vi "SCAN IM Stage Engine.vi"(0 "Notifier Name":string, 11 "COM Port":string[](array[string])) -> ()   [LabVIEW 2020]
uses:
  Stages Controls/Stage XY Control.ctl
  Stages Controls/Stage Status.ctl
  Stages Controls/Stage Notifier Element.ctl
  Stages Controls/Stage Actions.ctl
  <userlib>/Tango_DLL/Tango_DLL.lvlib
panel:
  out "Status":T1
  in  "Quit":bool
  in  "XY Control":T2
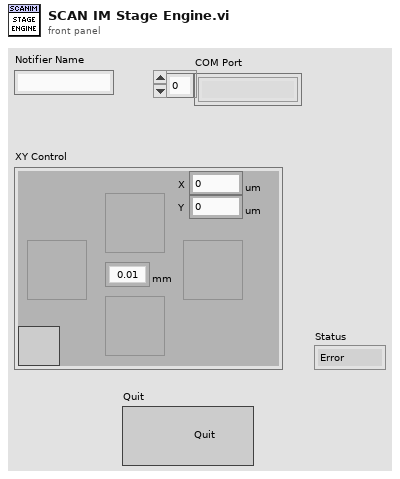
[diagram p1: front panel]
types:
  T1 = typedef "Stage Status.ctl" = enum16{"Error", "Abort", "Busy", "On Target"}
  T2 = typedef "Stage XY Control.ctl" = cluster{"Left":bool, "Right":bool, "Up":bool, "Down":bool, "Home":bool, "StageStep":enum16{"0.01", "0.02", "0.05", "0.1", "0.5", "1", "2", "5", "10", "20", "50", "100", "500", "1000", "2000", "5000"}, "Y":dbl, "X":dbl}
  T3 = typedef "Stage Notifier Element.ctl" = cluster{"Action":T4, "Axis":bool[], "Setpoint":dbl[], "Velocity":dbl, "Cmd Recvd?":bool, "Position":dbl[], "Status":T1, "Misc":variant}
  T4 = typedef "Stage Actions.ctl" = enum16{"Get Position", "MVR", "MOVE", "HALT", "ONTARGET", "ERROR", "REFERENCE", "INIT", "VELOCITY", "STATUS", "EXIT", "HOME", "ZEROPOS", "NANOPOS", "ANALOG", "QUIT"}
  T5 = cluster{"Left":bool, "Right":bool, "Up":bool, "Down":bool, "Home":bool, "StageStep":bool, "Y":bool, "X":bool}
  T6 = enum16{"0.01", "0.02", "0.05", "0.1", "0.5", "1", "2", "5", "10", "20", "50", "100", "500", "1000", "2000", "5000"}
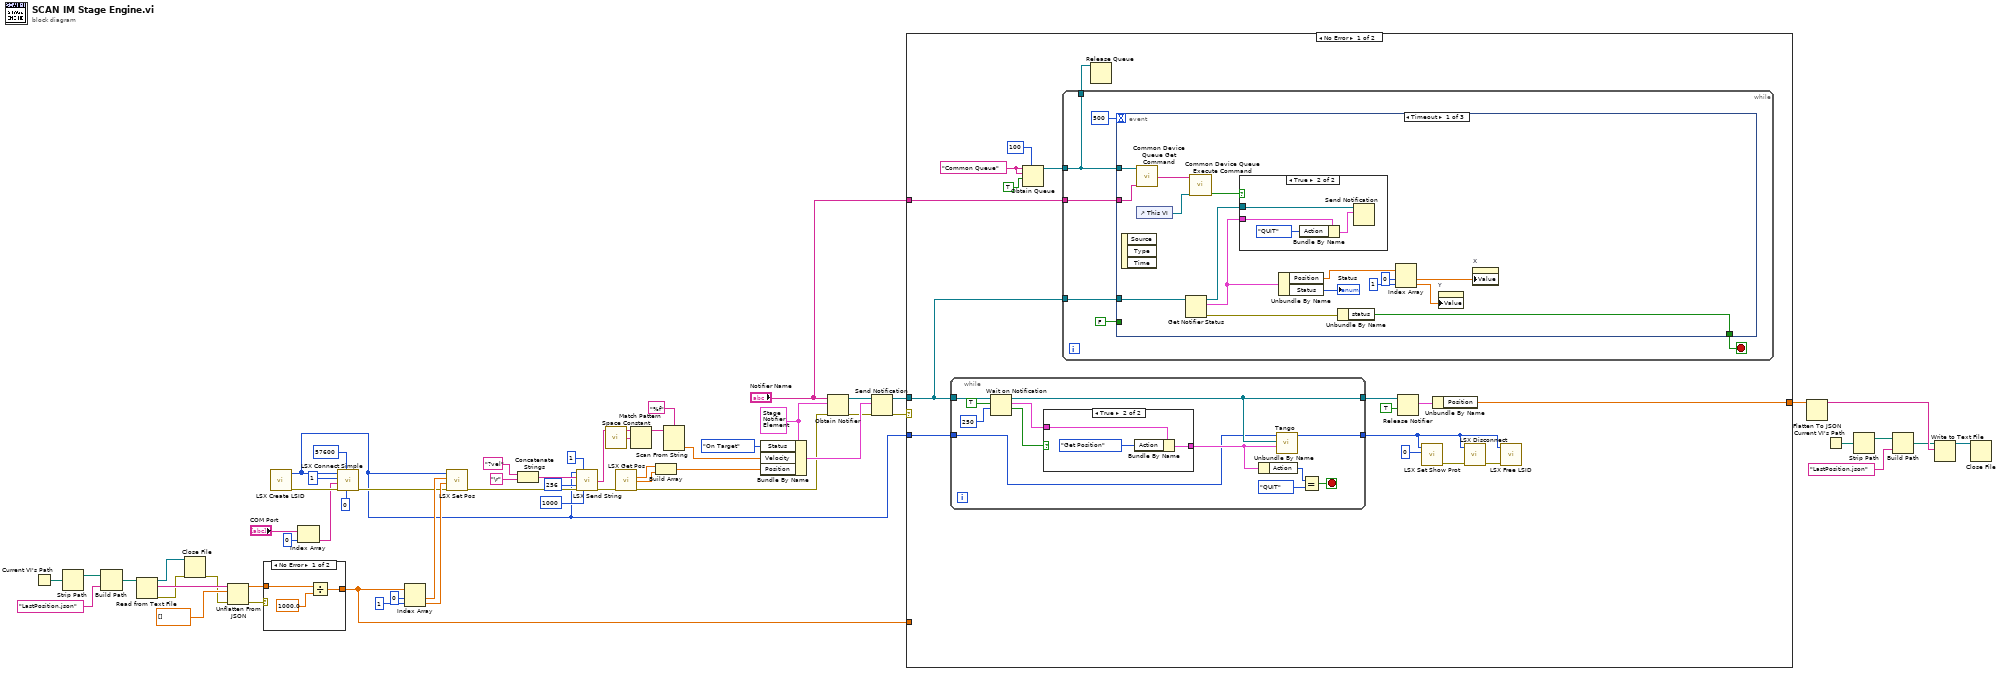
[diagram p0: block diagram]
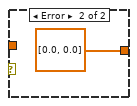
[diagram p2: hidden frame]
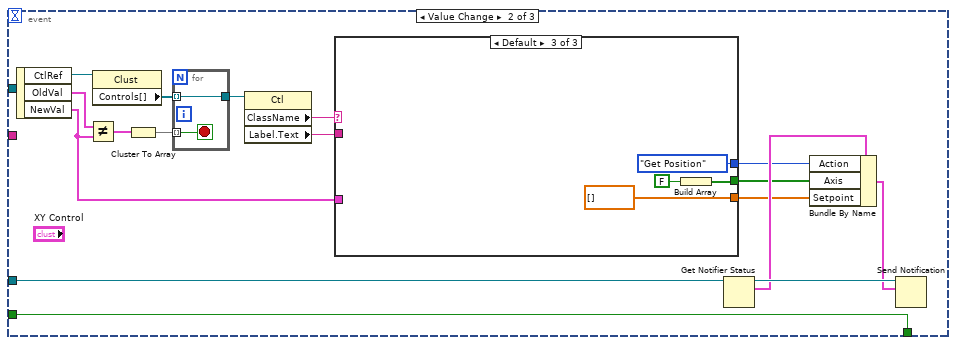
[diagram p5: hidden frame]
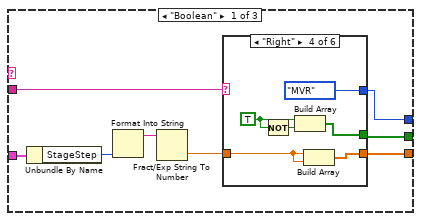
[diagram p6: hidden frame]
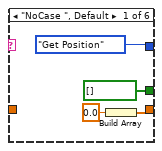
[diagram p7: hidden frame]
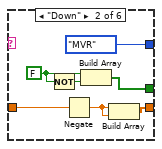
[diagram p8: hidden frame]
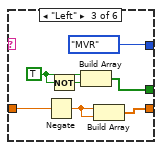
[diagram p9: hidden frame]
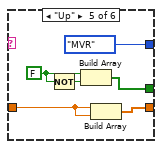
[diagram p10: hidden frame]
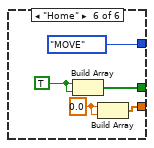
[diagram p11: hidden frame]
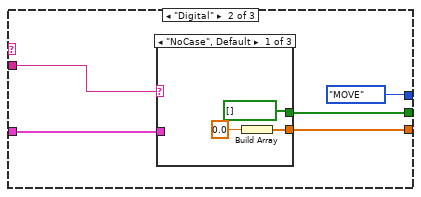
[diagram p12: hidden frame]
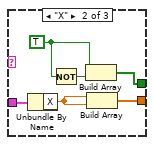
[diagram p13: hidden frame]
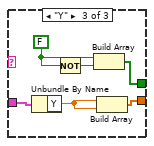
[diagram p14: hidden frame]
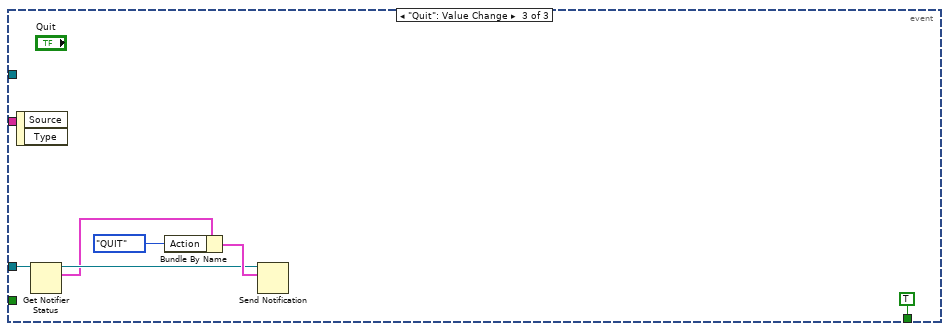
[diagram p15: hidden frame]
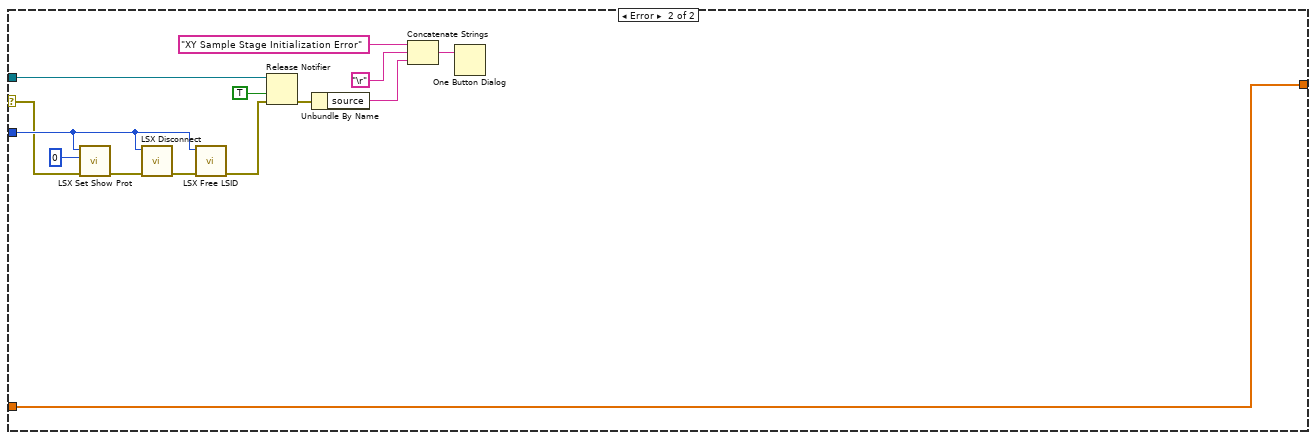
[diagram p16: hidden frame]
diagram:
  w56 = T3 {"Action"=enum."Get Position", "Axis"=[], "Setpoint"=[], "Velocity"=0.5, "Cmd Recvd?"=FALSE, "Position"=[], "Status"=enum."Abort", "Misc"=variant} ("Stage Status")
  n1 = Current VI's Path() -> (path=w39:path)
  n2 = Strip Path(path=w39) -> (stripped path=w38:path)  [unwired: 1 out]
  n3 = Build Path(base path=w38, name or relative path="LastPosition.json") -> (appended path=w36:path)
  n4 = Read from Text File(file (use dialog)=w36) -> (refnum out=w34:refnum<file>, text=w35:string, error out=w32:errorcluster)  [unwired: 3 in, 1 out]
  n5 = Close File(refnum=w34, error in=w32) -> (error out=w31:errorcluster)  [unwired: 1 out]
  n6 = Unflatten From JSON(JSON string=w35, type and defaults=dbl[] [], error in (no error)=w31) -> (value=w29:dbl[], error out=w30:errorcluster)  [unwired: 4 in]
  n7 = case shown="No Error" w30 {
    tunnel: w29 -> [w60 _]
    tunnel: [w58 dbl[] [0.0, 0.0]] -> w17
    frame No Error {
      n8 = Divide(x=w60, y=1000.0) -> (x/y=w58:dbl[])
    }
    frame Error {
    }
  }
  n9 = call <userlib>:"LSX Create LSID.vi"() -> ("error out"=w52:errorcluster, "plLSID out"=w3:i32)  [unwired: 9 in, 1 out]
  n10 = Index Array(array="COM Port", index=0) -> (element=w43:string)
  n11 = call <userlib>:"LSX Connect Simple.vi"("bAShowProt"=0, "lABaudRate"=57600, "error in (no error)"=w52, "pcAComName"=w43, "lAnInterfaceType"=1, "lLSID"=w3) -> ("error out"=w10:errorcluster)  [unwired: 3 in, 2 out]
  n12 = Index Array(array=w17, index #1=0 ("index"), index #2=1 ("index")) -> (element #1=w26:dbl, element #2=w25:dbl)
  n13 = call <userlib>:"LSX Set Pos.vi"("error in (no error)"=w10, "dY"=w25, "dX"=w26, "lLSID"=w3) -> ("error out"=w5:errorcluster)  [unwired: 6 in, 1 out]
  n14 = Concatenate Strings("?vel" ("pcStr"), "\r") -> (w11:string)
  n15 = call <userlib>:"LSX Send String.vi"("lLSID"=w3, "bReadLine"=1, "pcStr"=w11, "lMaxLen"=256, "error in (no error)"=w5, "lTimeOut"=1000) -> ("pcRet out"=w6:string, "error out"=w4:errorcluster)  [unwired: 6 in, 2 out]
  n16 = call <vilib>:"Space Constant.vi"() -> ("String"=w9:string)
  n17 = call <userlib>:"LSX Get Pos.vi"("error in (no error)"=w4) -> ("pdX out"=w48:dbl, "pdY out"=w47:dbl, "error out"=w42:errorcluster)  [unwired: 9 in, 3 out]
  n18 = Match Pattern(string=w6, regular expression=w9) -> (before substring=w8:string)  [unwired: 1 in, 3 out]
  n19 = Build Array(w48, w47) -> (w2:dbl[])
  n20 = Scan From String(format string="%f", input string=w8) -> (output 1=w1:dbl)  [unwired: 3 in, 3 out]
  n21 = Bundle By Name(cluster=w56, "Status"=Stage_Status."On Target", "Velocity"=w1, "Position"=w2) -> (w55:T3)
  n22 = Obtain Notifier(name (unnamed)="Notifier Name", notification data type=w56, error in (no error)=w42) -> (notifier out=w57:refnum<notifier>, error out=w46:errorcluster)  [unwired: 1 in, 1 out]
  n23 = Send Notification(notification=w55, notifier=w57, error in (no error)=w46) -> (notifier out=w54:refnum<notifier>, error out=w41:errorcluster)
  n24 = case shown="No Error" w41 {
    selector: w41 -> [_ w214]
    tunnel: w54 -> [w76 w219]
    tunnel: w3 -> [w70 w215]
    tunnel: "Notifier Name" -> [w64 _]
    tunnel: [w62 w212] -> w18
    tunnel: w17 -> [_ w212]
    frame No Error {
      w67 = "Common Queue" ("Unique Notifier Name")
      n25 = while {
        tunnel: w70 -> [w78]
        tunnel: [w89] -> w71
        tunnel: w76 -> [w86]
        tunnel: [w79] -> w75
        stop <- w88 stop-if-true
        n26 = Wait on Notification(notifier=w86, ignore previous (F)=TRUE, timeout in ms (-1)=250) -> (notifier out=w79:refnum<notifier>, notification=w81:T3, timed out?=w82:bool)  [unwired: 1 in, 1 out]
        n27 = case shown="True" w82 {
          tunnel: w81 -> [w90 w93]
          tunnel: [w90 w91] -> w80
          frame False {
          }
          frame True {
            n28 = Bundle By Name(cluster=w93, "Action"=Stage_Actions."Get Position") -> (w91:T3)
          }
        }
        n29 = Unbundle By Name(w80) -> ("Action"=w84:T4)
        n30 = call "Tango.vi"("Stage Action"=w80, "Scan IM Notifier"=w79, "Tango Handle"=w78) -> ("Tango Handle"=w89:i32)  [unwired: 8 in]
        n31 = Equal?(x=w84, y=Stage_Actions."QUIT") -> (x = y?=w88:bool)
      }
      n32 = Obtain Queue(max queue size (-1, unlimited)=100, name (unnamed)=w67, element data type=w67, create if not found? (T)=TRUE) -> (queue out=w66:refnum<queue>)  [unwired: 1 in, 2 out]
      n33 = while {
        tunnel: w76 -> [w97]
        tunnel: w66 -> [w96]
        tunnel: [w96] -> w65
        tunnel: w64 -> [w95]
        stop <- w98 stop-if-true
        n34 = event shown="[0] Timeout" {
          selector: _ -> [_ _ _]
          dyn-events: _ -> [_ _ _]
          timeout: 500 -> [_ _ _]
          tunnel: [w115 w120 TRUE ("status")] -> w98
          tunnel: w97 -> [w114 w130 w210]
          tunnel: w96 -> [w106 _ _]
          tunnel: w95 -> [w105 _ _]
          tunnel: FALSE ("status") -> [_ w120 _]
          event Timeout {
            n35 = event-data() -> ()  [unwired: 1 in, 3 out]
            n36 = call "Common Device Queue Get Command.vi"("Common Queue"=w106, "Notifier Name"=w105) -> ("Command"=w104:string)  [unwired: 12 in, 1 out]
            n37 = control-ref of="This VI"() -> (w103:refnum<vi>)
            n38 = Get Notifier Status(notifier=w114) -> (notifier out=w102:refnum<notifier>, current notification=w100:T3, error out=w113:errorcluster)  [unwired: 1 in, 2 out]
            n39 = call "Common Device Queue Execute Command.vi"("Common Command"=w104, "VI Refnum"=w103) -> ("Quit?"=w107:bool)  [unwired: 12 in, 1 out]
            n40 = case shown="True" w107 {
              tunnel: w102 -> [_ w119]
              tunnel: w100 -> [_ w118]
              frame False {
              }
              frame True {
                n41 = Bundle By Name(cluster=w118, "Action"=Stage_Actions."QUIT") -> (w117:T3)
                n42 = Send Notification(notification=w117, notifier=w119) -> ()  [unwired: 1 in, 2 out]
              }
            }
            n43 = Unbundle By Name(w100) -> ("Position"=w101:dbl[], "Status"=→"Status":T1)
            n44 = Unbundle By Name(w113) -> ("status"=w115:bool)
            n45 = Index Array(array=w101, index #1=0 ("index"), index #2=1 ("index")) -> (element #1=w111:dbl, element #2=w110:dbl)
            n46 = property on="Y" class="DigNum (strict)"("Value"=w110) -> ()  [unwired: 2 in, 2 out]
            n47 = property on="X" class="DigNum (strict)"("Value"=w111) -> ()  [unwired: 2 in, 2 out]
          }
          event Value Change {
            n48 = event-data() -> ("CtlRef"=w135:refnum<vi>, "OldVal"=w136:T2, "NewVal"=w124:T2)  [unwired: 1 in]
            n49 = Not Equal?(x=w136, y=w124) -> (x != y?=w134:T5)
            n50 = property class="Clust"(reference=w135) -> ("Controls[]"=w132:refnum<vi>[])  [unwired: 1 in, 2 out]
            n51 = Cluster To Array(cluster=w134) -> (array=w133:bool[])
            n52 = for {
              tunnel: w133 -> [w205] mode=indexing
              tunnel: [w204] -> w131
              tunnel: w132 -> [w204] mode=indexing
              stop <- w205 stop-if-true
            }
            n53 = property class="Ctl"(reference=w131) -> ("ClassName"=w126:string, "Label.Text"=w125:string)  [unwired: 1 in, 2 out]
            n54 = case shown="Default" w126 {
              tunnel: w124 -> [w144 w183 _]
              tunnel: w125 -> [w139 w184 _]
              tunnel: [w140 w182 dbl[] []] -> w122
              tunnel: [w141 w181 w202] -> w123
              tunnel: [w137 Stage_Actions."MOVE" ("Action") Stage_Actions."Get Position" ("Action")] -> w121
              frame "Boolean" {
                n55 = Unbundle By Name(w144) -> ("StageStep"=w142:T6)
                n56 = Format Into String(w142) -> (resulting string=w143:string)  [unwired: 3 in, 1 out]
                n57 = Fract/Exp String To Number(string=w143) -> (number=w138:dbl)  [unwired: 3 in, 1 out]
                n58 = case shown="\"Right\"" w139 {
                  tunnel: [w146 w151 w158 w165 w171 w177] -> w140
                  tunnel: [bool[] [] w152 w159 w166 w172 w179] -> w141
                  tunnel: w138 -> [_ w155 w162 w164 w170 _]
                  tunnel: [Stage_Actions."Get Position" ("Action") Stage_Actions."MVR" ("Action") Stage_Actions."MVR" ("Action") Stage_Actions."MVR" ("Action") Stage_Actions."MVR" ("Action") Stage_Actions."MOVE" ("Action")] -> w137
                  frame "NoCase ", Default {
                    n59 = Build Array(0.0) -> (w146:dbl[])
                  }
                  frame "Down" {
                    w153 = FALSE
                    n60 = Not(x=w153) -> (.not. x?=w154:bool)
                    n61 = Negate(x=w155) -> (-x=w150:dbl)
                    n62 = Build Array(w153, w154) -> (w152:bool[])
                    n63 = Build Array(w150, w150) -> (w151:dbl[])
                  }
                  frame "Left" {
                    w160 = TRUE
                    n64 = Negate(x=w162) -> (-x=w157:dbl)
                    n65 = Not(x=w160) -> (.not. x?=w161:bool)
                    n66 = Build Array(w160, w161) -> (w159:bool[])
                    n67 = Build Array(w157, w157) -> (w158:dbl[])
                  }
                  frame "Right" {
                    w167 = TRUE
                    n68 = Not(x=w167) -> (.not. x?=w168:bool)
                    n69 = Build Array(w167, w168) -> (w166:bool[])
                    n70 = Build Array(w164, w164) -> (w165:dbl[])
                  }
                  frame "Up" {
                    w173 = FALSE
                    n71 = Not(x=w173) -> (.not. x?=w174:bool)
                    n72 = Build Array(w173, w174) -> (w172:bool[])
                    n73 = Build Array(w170, w170) -> (w171:dbl[])
                  }
                  frame "Home" {
                    w176 = 0.0
                    w178 = TRUE
                    n74 = Build Array(w178, w178) -> (w179:bool[])
                    n75 = Build Array(w176, w176) -> (w177:dbl[])
                  }
                }
              }
              frame "Digital" {
                n76 = case shown="\"NoCase\", Default" w184 {
                  tunnel: [bool[] [] w192 w197] -> w181
                  tunnel: w183 -> [_ w191 w196]
                  tunnel: [w185 w190 w195] -> w182
                  frame "NoCase", Default {
                    n77 = Build Array(0.0 ("Y axis (mm)")) -> (w185:dbl[])
                  }
                  frame "X" {
                    w193 = TRUE
                    n78 = Unbundle By Name(w191) -> ("X"=w189:dbl)
                    n79 = Not(x=w193) -> (.not. x?=w188:bool)
                    n80 = Build Array(w193, w188) -> (w192:bool[])
                    n81 = Build Array(w189, w189) -> (w190:dbl[])
                  }
                  frame "Y" {
                    w199 = FALSE
                    n82 = Unbundle By Name(w196) -> ("Y"=w194:dbl)
                    n83 = Not(x=w199) -> (.not. x?=w198:bool)
                    n84 = Build Array(w199, w198) -> (w197:bool[])
                    n85 = Build Array(w194, w194) -> (w195:dbl[])
                  }
                }
              }
              frame Default {
                n86 = Build Array(FALSE) -> (w202:bool[])
              }
            }
            n87 = Get Notifier Status(notifier=w130) -> (notifier out=w129:refnum<notifier>, current notification=w128:T3)  [unwired: 1 in, 3 out]
            n88 = Bundle By Name(cluster=w128, "Action"=w121, "Axis"=w123, "Setpoint"=w122) -> (w127:T3)
            n89 = Send Notification(notification=w127, notifier=w129) -> ()  [unwired: 1 in, 2 out]
          }
          event "Quit": Value Change {
            n90 = event-data() -> ()  [unwired: 1 in, 2 out]
            n91 = Get Notifier Status(notifier=w210) -> (notifier out=w208:refnum<notifier>, current notification=w206:T3)  [unwired: 1 in, 3 out]
            n92 = Bundle By Name(cluster=w206, "Action"=Stage_Actions."QUIT") -> (w211:T3)
            n93 = Send Notification(notification=w211, notifier=w208) -> ()  [unwired: 1 in, 2 out]
          }
        }
      }
      n94 = Release Queue(queue=w65) -> ()  [unwired: 2 in, 3 out]
      n95 = Release Notifier(notifier=w75, force destroy? (F)=TRUE) -> (last notification=w63:T3)  [unwired: 1 in, 2 out]
      n96 = call <userlib>:"LSX Set Show Prot.vi"("bShowProt"=0, "lLSID"=w71) -> ("error out"=w73:errorcluster)  [unwired: 8 in, 1 out]
      n97 = Unbundle By Name(w63) -> ("Position"=w62:dbl[])
      n98 = call <userlib>:"LSX Disconnect.vi"("error in (no error)"=w73, "lLSID"=w71) -> ("error out"=w74:errorcluster)  [unwired: 8 in, 1 out]
      n99 = call <userlib>:"LSX Free LSID.vi"("error in (no error)"=w74, "lLSID"=w71) -> ()  [unwired: 8 in, 2 out]
    }
    frame Error {
      n100 = call <userlib>:"LSX Set Show Prot.vi"("error in (no error)"=w214, "bShowProt"=0, "lLSID"=w215) -> ("error out"=w217:errorcluster)  [unwired: 7 in, 1 out]
      n101 = call <userlib>:"LSX Disconnect.vi"("error in (no error)"=w217, "lLSID"=w215) -> ("error out"=w218:errorcluster)  [unwired: 8 in, 1 out]
      n102 = call <userlib>:"LSX Free LSID.vi"("error in (no error)"=w218, "lLSID"=w215) -> ("error out"=w213:errorcluster)  [unwired: 8 in, 1 out]
      n103 = Release Notifier(notifier=w219, force destroy? (F)=TRUE, error in (no error)=w213) -> (error out=w224:errorcluster)  [unwired: 2 out]
      n104 = Unbundle By Name(w224) -> ("source"=w221:string)
      n105 = Concatenate Strings("XY Sample Stage Initialization Error", "\r", w221) -> (w220:string)
      n106 = One Button Dialog(message=w220) -> ()  [unwired: 1 in, 1 out]
    }
  }
  n107 = Flatten To JSON(anything=w18) -> (JSON string=w23:string)  [unwired: 2 in, 1 out]
  n108 = Current VI's Path() -> (path=w19:path)
  n109 = Strip Path(path=w19) -> (stripped path=w20:path)  [unwired: 1 out]
  n110 = Build Path(base path=w20, name or relative path="LastPosition.json") -> (appended path=w22:path)
  n111 = Write to Text File(file (use dialog)=w22, text=w23) -> (refnum out=w24:refnum<file>)  [unwired: 2 in, 2 out]
  n112 = Close File(refnum=w24) -> ()  [unwired: 1 in, 2 out]
